vi "Get SshHostKeyPolicy.vi"(8 "error in (no error)":errorcluster, 11 "SessionOptions-SCP in":refnum<class "SessionOptions-SCP.lvclass">) -> (0 "error out":errorcluster, 2 "SshHostKeyPolicy":T1=1 items=["Check", "GiveUpSecurityAndAcceptAny", "AcceptNew"], 3 "SessionOptions-SCP out":refnum<class "SessionOptions-SCP.lvclass">)   [LabVIEW 2015, in "SessionOptions-SCP.lvclass"]
uses:
  SessionOptions-SCP.lvclass
  SSHHostKeyPolicy.ctl
  SessionOptions-SCP.lvclass/SessionOptions-SCP.ctl
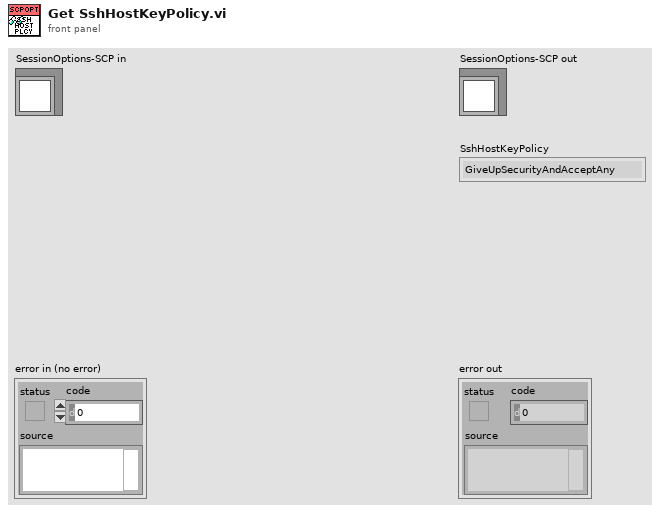
[diagram p1: front panel]
types:
  T1 = typedef "SessionOptions-SCP.lvclass/SSHHostKeyPolicy.ctl" = i32
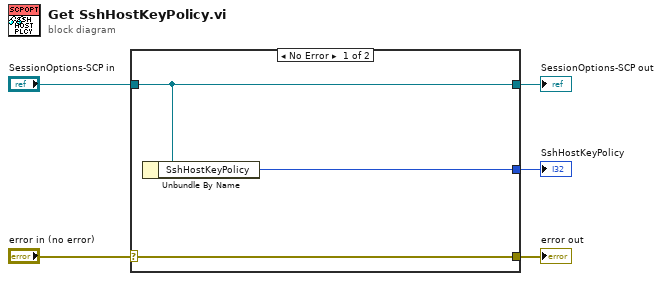
[diagram p0: block diagram]
diagram:
  n1 = case shown="No Error" "error in (no error)" {
    selector: "error in (no error)" -> [w8 w9]
    tunnel: [w8 w9] -> w4
    tunnel: [w7 w10] -> w2
    tunnel: "SessionOptions-SCP in" -> [w7 w10]
    tunnel: [w6 _] -> w1
    frame No Error {
      n2 = Unbundle By Name(w7) -> ("SshHostKeyPolicy"=w6:T1)
    }
    frame Error {
    }
  }
  "error out" <- w4
  "SessionOptions-SCP out" <- w2
  "SshHostKeyPolicy" <- w1
